vi "Zapis_ustawien_AI.vi"(8 "error in (no error)":errorcluster, 10 "Referencje Array":refnum<vi>[](array[refnum]), 11 "Plik konf in":path=path "D:/Marek/Dysk Google/Projekty LabVIEW/! Rudpol/Program/Konfiguracja/AI_Konfiguracja.txt") -> (0 "error out":errorcluster, 3 "Plik konf out":path)   [LabVIEW 2014]
doc: "Zapisuje ustawienia kana丑w AI do pliku\nAI_Konfiguracja.txt"
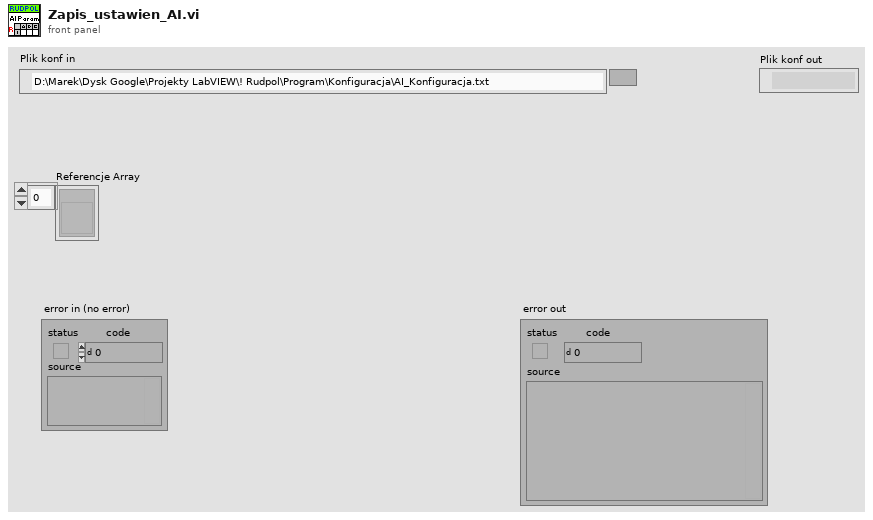
[diagram p1: front panel]
types:
  T1 = enum16{"open", "replace", "create", "open or create", "replace or create", "replace or create with confirmation"}
  T2 = typedef "AI_parametry.ctl" = cluster{"Numer":u8, "Opis":string, "Zakres":enum16{"1000V", "300V", "30V", "3V", "0,3V"}, "Filtr":bool, "Typ pomiaru":enum16{"Wartoœæ œrednia", "Œrednia wyprostowana", "Wartoœæ skuteczna"}, "Aktywny":bool, "Wartoœæ":T3}
  T3 = typedef "AI_wartosc.ctl" = cluster{"X":string, "[ ]":string, "trans X":dbl, "trans U":dbl, "Z tabeli":bool, "Opis":string}
  T4 = enum16{"Wartoœæ œrednia", "Œrednia wyprostowana", "Wartoœæ skuteczna"}
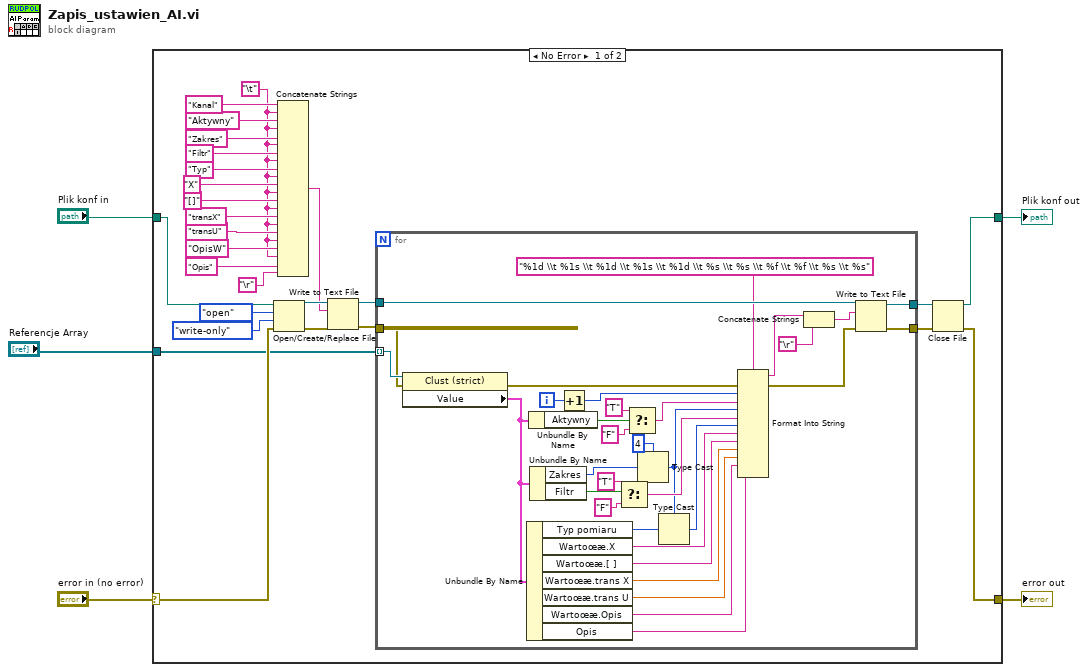
[diagram p0: block diagram]
diagram:
  n1 = case shown="No Error" "error in (no error)" {
    selector: "error in (no error)" -> [w28 w67]
    tunnel: [w7 w67] -> w4
    tunnel: "Plik konf in" -> [w30 w66]
    tunnel: [w29 w66] -> w3
    tunnel: "Referencje Array" -> [w8 _]
    frame No Error {
      w10 = "\t"
      n2 = Open/Create/Replace File(file path (use dialog)=w30, error in=w28, operation (0:open)=T1."open", access (0:read/write)=enum16{"read/write", "read-only", "write-only"}."write-only") -> (refnum out=w25:refnum<file>, error out=w24:errorcluster)  [unwired: 2 in, 1 out]
      n3 = Concatenate Strings("Kanal" ("string"), w10, "Aktywny" ("string"), w10, "Zakres" ("string"), w10, "Filtr" ("string"), w10, "Typ" ("string"), w10, "X" ("string"), w10, "[]" ("string"), w10, "transX" ("string"), w10, "transU" ("string"), w10, "OpisW" ("string"), w10, "Opis" ("string"), "\r") -> (w9:string)
      n4 = Write to Text File(file (use dialog)=w25, text=w9, error in=w24) -> (refnum out=w22:refnum<file>, error out=w23:errorcluster)  [unwired: 1 in, 1 out]
      n5 = for {
        tunnel: [w65] -> w27
        tunnel: [w64] -> w26
        tunnel: w23 -> [w61]
        tunnel: w22 -> [w63]
        tunnel: w8 -> [w62] mode=indexing
        i -> [w34]
        n6 = property class="Clust (strict)"(reference=w62, error in=w61) -> (error out=w59:errorcluster, "Value"=w49:T2)  [unwired: 1 out]
        n7 = Unbundle By Name(w49) -> ("Typ pomiaru"=w40:T4, "Wartoœæ.X"=w48:string, "Wartoœæ.[ ]"=w47:string, "Wartoœæ.trans X"=w46:dbl, "Wartoœæ.trans U"=w45:dbl, "Wartoœæ.Opis"=w44:string, "Opis"=w43:string)
        n8 = Unbundle By Name(w49) -> ("Aktywny"=w57:bool)
        n9 = Unbundle By Name(w49) -> ("Zakres"=w41:enum16{"1000V", "300V", "30V", "3V", "0,3V"}, "Filtr"=w52:bool)
        n10 = Increment(x=w34) -> (x+1=w33:i32)
        n11 = Select(t="T" ("string"), s=w52, f="F" ("string")) -> (s? t:f=w50:string)
        n12 = Select(t="T" ("string"), s=w57, f="F" ("string")) -> (s? t:f=w55:string)
        n13 = Type Cast(type=u16 4 ("upper limit"), x=w41) -> (*(type *) &x=w38:u16)
        n14 = Type Cast(type=w38, x=w40) -> (*(type *) &x=w39:u16)
        n15 = Format Into String(format string="%1d \\t %1s \\t %1d \\t %1s \\t %1d \\t %s \\t %s \\t %f \\t %f \\t %s \\t %s", error in=w59, w33, w55, w38, w50, w39, w48, w47, w46, w45, w44, w43) -> (resulting string=w36:string, error out=w58:errorcluster)  [unwired: 1 in]
        n16 = Concatenate Strings(w36, "\r") -> (w37:string)
        n17 = Write to Text File(file (use dialog)=w63, text=w37, error in=w58) -> (refnum out=w64:refnum<file>, error out=w65:errorcluster)  [unwired: 1 in, 1 out]
      }
      n18 = Close File(refnum=w26, error in=w27) -> (path=w29:path, error out=w7:errorcluster)
    }
    frame Error {
    }
  }
  "error out" <- w4
  "Plik konf out" <- w3
